vi "Logging Edit Tree Item.vi"() -> ()   [LabVIEW 2012]
uses:
  Log Entry.ctl
  Log Value Type.ctl
  Log Value Cluster.ctl
  femtoRoboLib.lvlib
panel:
  in  "Log Entry":T1
  in  "TreeRef":refnum<vi>
  out "TreeRef":refnum<vi>
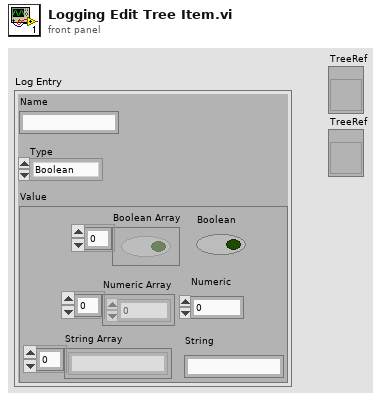
[diagram p1: front panel]
types:
  T1 = typedef "femtoRoboLib.lvlib/Log Entry.ctl" = cluster{"Name":string, "Type":T2, "Value":T3}
  T2 = typedef "femtoRoboLib.lvlib/Log Value Type.ctl" = enum16{"Boolean", "Numeric", "String", "Boolean Array", "Numeric Array", "String Array"}
  T3 = typedef "femtoRoboLib.lvlib/Log Value Cluster.ctl" = cluster{"Boolean Array":bool[], "Boolean":bool, "Numeric Array":dbl[], "Numeric":dbl, "String Array":string[], "String":string}
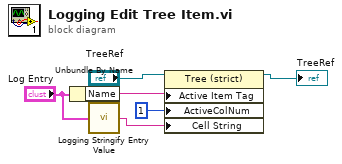
[diagram p0: block diagram]
diagram:
  n1 = Unbundle By Name("Log Entry") -> ("Name"=w3:string)
  n2 = call "Logging Stringify Entry Value.vi"("Entry"="Log Entry") -> ("String"=w1:string)
  n3 = property class="Tree (strict)"(reference="TreeRef", "Active Item Tag"=w3, "ActiveColNum"=1 ("Active Cell:Active Column Number"), "Cell String"=w1) -> (reference out=→"TreeRef":refnum<vi>)  [unwired: 1 in, 1 out]
